vi "resetView.vi"(8 "error in (no error)":errorcluster, 11 "TransactionListUIAdapter in":refnum<class "TransactionListUIAdapter.lvclass">) -> (0 "error out":errorcluster, 3 "TransactionListUIAdapter out":refnum<class "TransactionListUIAdapter.lvclass">)   [LabVIEW 2020, in "TransactionListUIAdapter.lvclass"]
uses:
  TransactionListUIAdapter.lvclass
  AbstractMultiColumnListBoxAdapter/AbstractMultiColumnListBoxAdapter.lvclass
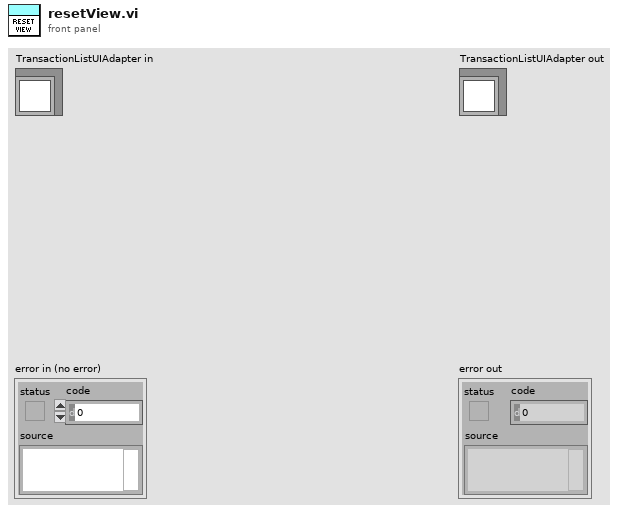
[diagram p1: front panel]
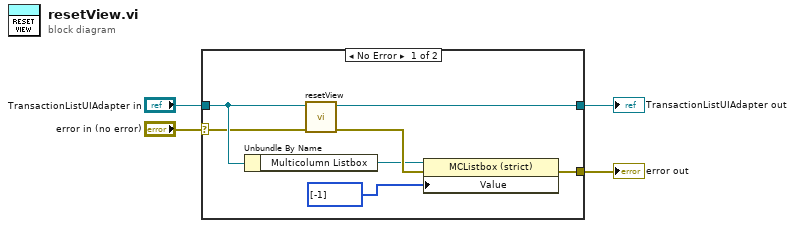
[diagram p0: block diagram]
diagram:
  n1 = case shown="No Error" "error in (no error)" {
    selector: "error in (no error)" -> [w6 w12]
    tunnel: [w11 w13] -> w4
    tunnel: [w9 w12] -> w3
    tunnel: "TransactionListUIAdapter in" -> [w8 w13]
    frame No Error {
      n2 = Unbundle By Name(w8) -> ("Multicolumn Listbox"=w7:refnum<vi>)
      n3 = call-parent "resetView.vi"("error in (no error)"=w6, "AbstractMultiColumnListBoxAdapter in"=w8) -> ("error out"=w10:errorcluster, "AbstractMultiColumnListBoxAdapter out"=w11:refnum<class "TransactionListUIAdapter.lvclass">)  [unwired: 8 in]
      n4 = property class="MCListbox (strict)"(reference=w7, error in=w10, "Value"=i32[] [-1]) -> (error out=w9:errorcluster)  [unwired: 1 out]
    }
    frame Error {
    }
  }
  "error out" <- w3
  "TransactionListUIAdapter out" <- w4
